vi "Independent Component Analysis.vi"() -> ()   [LabVIEW 2023]
doc: "This example shows how to perform independent components analysis on a multivariate time series with the TSA Independent Component Analysis VI.\n\n<b>Instructions:</b>\n1) Run this VI.\n2) Configure signal simulation settings.\n3) Observe the recovered signals from ICA. \n4) To know the values of the mixing matrix A, browse the Block Diagram."
uses:
  <vilib>/Analysis/baseanly.llb/Real A x B.vi
  <vilib>/addons/Time Series Analysis/Statistical Analysis.llb/TSA Independent Component Analysis (Array).vi
  <vilib>/Analysis/NI_AALBase.lvlib
  <vilib>/addons/_Advanced Signal Processing/NI_AdvSigProcTSA.lvlib
panel:
  in  "stop":bool
  in  "Noise 2":dbl(slide)=0.025 scale=0.0..0.4
  in  "Noise 1":dbl(slide)=0.025 scale=0.0..0.4
  in  "Phase 2":dbl(slide)=90.0 scale=0.0..180.0
  in  "Phase 1":dbl(slide)=30.0 scale=0.0..180.0
  in  "Freq 2":dbl(slide)=0.004 scale=0.001..0.1 scale format="%#.2f"
  in  "Freq 1":dbl(slide)=0.013122448979591837 scale=0.001..0.1 scale format="%#.2f"
  in  "Amp 2":dbl(slide)=2.0 scale=0.0..5.0
  in  "Amp 1":dbl(slide)=1.0 scale=0.0..5.0
  in  "Signal Type":u16(ring) items=["sine + triangular", "sine + square", "sine + sawtooth", "triangular + square"]
  in  "Method":u16(ring)=1 items=["Matrix Pencil ICA", "Fast ICA"]
  out "Recovered Signals":dbl[][](graph)
  out "Mixed Signals (x = As)":dbl[][](graph)
  out "Original Signals":dbl[][](graph)
  # "Overview: Shows how to perform independent components analysis on a multivariate time series with the TSA Independent Component Analysis VI.\nRequirements: LabVIEW Full Development System, Advanced Signal Processing Toolkit\nInstructions: \n1. Run this VI.\n2. Configure signal simulation settings.\n3. Observe the recovered signals from ICA. \n4. To know the values of the mixing matrix A, browse the block diagram.\n5. Click Stop to stop the VI."
  # "Signal Simulation"
  # "Signal Mixing Simulation"
  # "ICA"
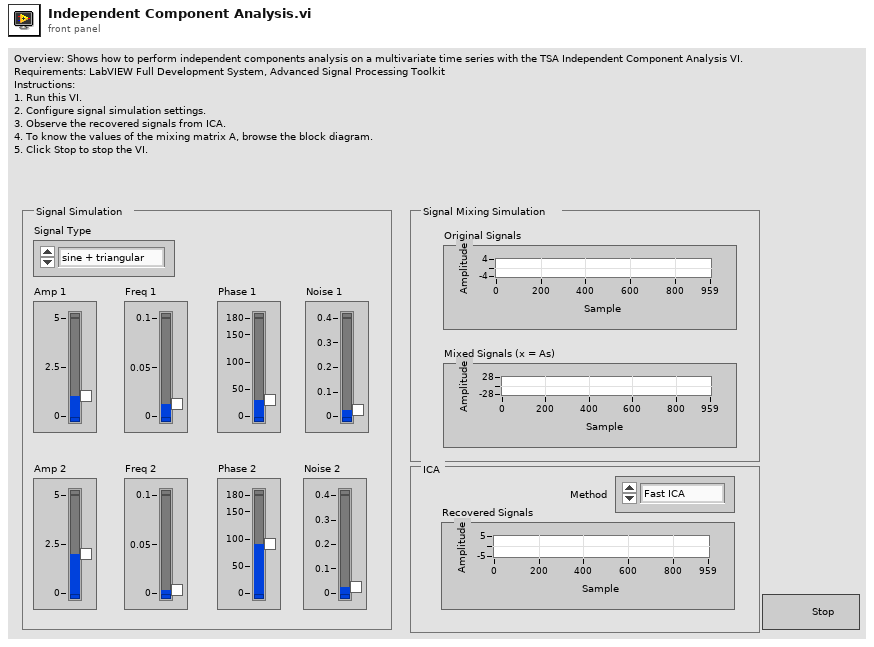
[diagram p1: front panel]
types:
  T1 = typedef "NI_Matrix.lvlib/RealMatrix.ctl" = dbl[][]
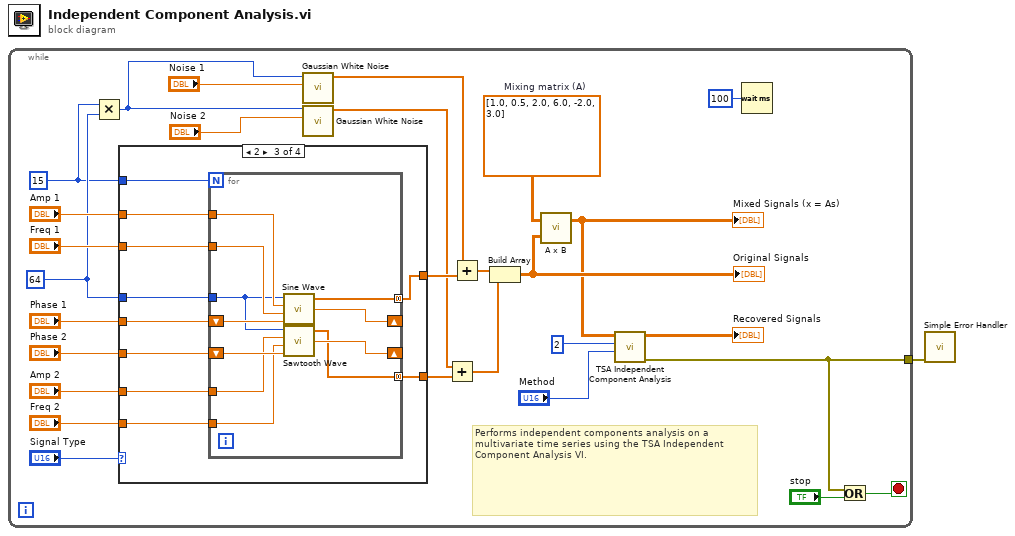
[diagram p0: block diagram]
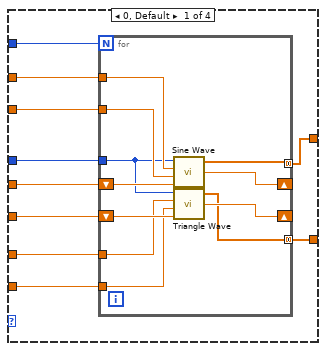
[diagram p2: hidden frame]
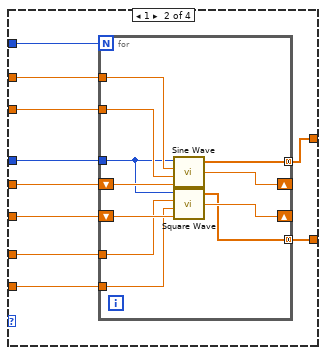
[diagram p3: hidden frame]
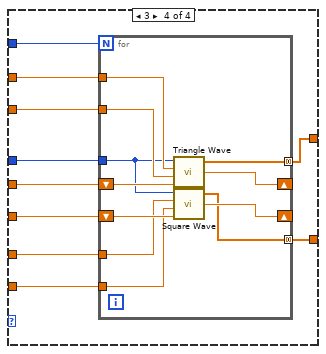
[diagram p4: hidden frame]
diagram:
  n1 = while {
    tunnel: [w2] -> w1
    stop <- w5 stop-if-true
    w29 = dbl[][] [[1.0, 0.5], [2.0, 6.0], [-2.0, 3.0]]  # Mixing matrix (A)
    w15 = 64 ("samples")
    w14 = 15
    # "Performs independent components analysis on a multivariate time series using the TSA Independent Component Analysis VI."
    n2 = Multiply(x=w14, y=w15) -> (x*y=w13:i32)
    n3 = case shown="2" "Signal Type" {
      tunnel: [w31 w52 w73 w94] -> w27
      tunnel: [w30 w51 w72 w93] -> w26
      tunnel: "Freq 2" -> [w39 w60 w81 w102]
      tunnel: "Amp 2" -> [w38 w59 w80 w101]
      tunnel: "Freq 1" -> [w37 w58 w79 w100]
      tunnel: "Amp 1" -> [w36 w57 w78 w99]
      tunnel: w14 -> [w32 w54 w74 w95]
      tunnel: "Phase 1" -> [w35 w56 w77 w98]
      tunnel: "Phase 2" -> [w34 w55 w76 w97]
      tunnel: w15 -> [w33 w53 w75 w96]
      frame 0, Default {
        n4 = for {
          N: w32 -> [_]
          shift-right: [w49] -> _
          shift-left: w35 -> [w50]
          shift-right: [w47] -> _
          shift-left: w34 -> [w48]
          tunnel: w38 -> [w46]
          tunnel: w39 -> [w45]
          tunnel: w37 -> [w44]
          tunnel: w36 -> [w43]
          tunnel: w33 -> [w42]
          tunnel: [w41] -> w31 mode=concatenating
          tunnel: [w40] -> w30 mode=concatenating
          n5 = call <vilib>:"Sine Wave.vi"("samples"=w42, "amplitude"=w43, "frequency"=w44, "phase in"=w50) -> ("sine wave"=w41:dbl[], "phase out"=w49:dbl)  [unwired: 1 in, 1 out]
          n6 = call <vilib>:"Triangle Wave.vi"("samples"=w42, "amplitude"=w46, "frequency"=w45, "phase in"=w48) -> ("triangle wave"=w40:dbl[], "phase out"=w47:dbl)  [unwired: 1 in, 1 out]
        }
      }
      frame 1 {
        n7 = for {
          N: w54 -> [_]
          shift-right: [w70] -> _
          shift-left: w56 -> [w71]
          shift-right: [w68] -> _
          shift-left: w55 -> [w69]
          tunnel: w59 -> [w67]
          tunnel: w60 -> [w66]
          tunnel: w58 -> [w65]
          tunnel: w57 -> [w64]
          tunnel: w53 -> [w63]
          tunnel: [w62] -> w52 mode=concatenating
          tunnel: [w61] -> w51 mode=concatenating
          n8 = call <vilib>:"Sine Wave.vi"("samples"=w63, "amplitude"=w64, "frequency"=w65, "phase in"=w71) -> ("sine wave"=w62:dbl[], "phase out"=w70:dbl)  [unwired: 1 in, 1 out]
          n9 = call <vilib>:"Square Wave.vi"("samples"=w63, "amplitude"=w67, "frequency"=w66, "phase in"=w69) -> ("square wave"=w61:dbl[], "phase out"=w68:dbl)  [unwired: 2 in, 1 out]
        }
      }
      frame 2 {
        n10 = for {
          N: w74 -> [_]
          shift-right: [w91] -> _
          shift-left: w77 -> [w92]
          shift-right: [w89] -> _
          shift-left: w76 -> [w90]
          tunnel: w80 -> [w88]
          tunnel: w81 -> [w87]
          tunnel: w79 -> [w86]
          tunnel: w78 -> [w85]
          tunnel: w75 -> [w84]
          tunnel: [w83] -> w73 mode=concatenating
          tunnel: [w82] -> w72 mode=concatenating
          n11 = call <vilib>:"Sine Wave.vi"("samples"=w84, "amplitude"=w85, "frequency"=w86, "phase in"=w92) -> ("sine wave"=w83:dbl[], "phase out"=w91:dbl)  [unwired: 1 in, 1 out]
          n12 = call <vilib>:"Sawtooth Wave.vi"("samples"=w84, "amplitude"=w88, "frequency"=w87, "phase in"=w90) -> ("sawtooth wave"=w82:dbl[], "phase out"=w89:dbl)  [unwired: 1 in, 1 out]
        }
      }
      frame 3 {
        n13 = for {
          N: w95 -> [_]
          shift-right: [w112] -> _
          shift-left: w98 -> [w113]
          shift-right: [w110] -> _
          shift-left: w97 -> [w111]
          tunnel: w101 -> [w109]
          tunnel: w102 -> [w108]
          tunnel: w100 -> [w107]
          tunnel: w99 -> [w106]
          tunnel: w96 -> [w105]
          tunnel: [w104] -> w94 mode=concatenating
          tunnel: [w103] -> w93 mode=concatenating
          n14 = call <vilib>:"Triangle Wave.vi"("samples"=w105, "amplitude"=w106, "frequency"=w107, "phase in"=w113) -> ("triangle wave"=w104:dbl[], "phase out"=w112:dbl)  [unwired: 1 in, 1 out]
          n15 = call <vilib>:"Square Wave.vi"("samples"=w105, "amplitude"=w109, "frequency"=w108, "phase in"=w111) -> ("square wave"=w103:dbl[], "phase out"=w110:dbl)  [unwired: 2 in, 1 out]
        }
      }
    }
    n16 = call <vilib>:"Gaussian White Noise.vi"("standard deviation"="Noise 1", "samples"=w13) -> ("Gaussian noise pattern"=w9:dbl[])  [unwired: 8 in, 1 out]
    n17 = call <vilib>:"Gaussian White Noise.vi"("standard deviation"="Noise 2", "samples"=w13) -> ("Gaussian noise pattern"=w7:dbl[])  [unwired: 8 in, 1 out]
    n18 = Add(x=w7, y=w26) -> (x+y=w8:dbl[])
    n19 = Add(x=w9, y=w27) -> (x+y=w10:dbl[])
    n20 = Build Array(w10, w8) -> (w25:dbl[][])
    "Original Signals" <- w25
    n21 = call-poly <vilib>:"A x B.vi"("B"=w25, "A"=w29) -> ("A x B"=w24:T1)  [unwired: 1 out]
    "Mixed Signals (x = As)" <- w24
    n22 = call-poly <vilib>:"TSA Independent Component Analysis.vi"("ICA method"="Method", "number of IC"=2 ("# of IC"), "Xt"=w24) -> ("error out"=w2:errorcluster, "Xt out"=→"Recovered Signals":dbl[][])  [unwired: 1 in, 6 out]
    n23 = Wait (ms)(milliseconds to wait=u32 100 ("millisecond multiple")) -> ()  [unwired: 1 out]
    n24 = Or(x=w2, y="stop") -> (x .or. y?=w5:bool)
  }
  n25 = call <vilib>:"Simple Error Handler.vi"("error in (no error)"=w1) -> ()  [unwired: 1 in, 8 out]
